vi "DAQ_Power_postwrite.vi"(9 "stop":bool) -> ()   [LabVIEW 2020]
uses:
  <vilib>/Utility/error.llb/DialogType.ctl
  <vilib>/ULx/Create Channel.llb/ULx Create Channel (AI-Voltage-Basic).vi
  <vilib>/ULx/Timing.llb/ULx Timing (Sample Clock).vi
  <vilib>/ULx/Read.llb/ULx Read (Analog 1D Wfm NChan NSamp).vi
panel:
  out "Power Graph":waveform(dbl)[](graph)
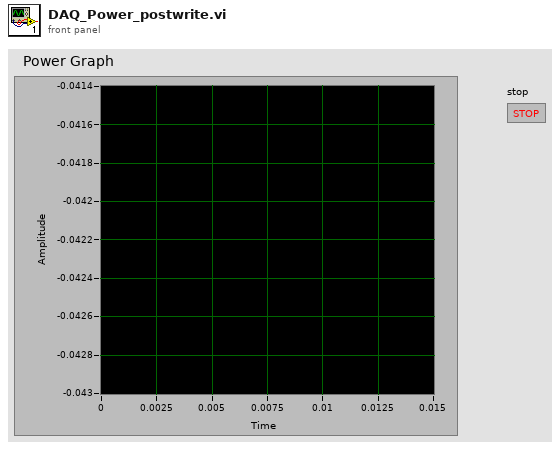
[diagram p1: front panel]
types:
  T1 = typedef "DialogType.ctl" = u16
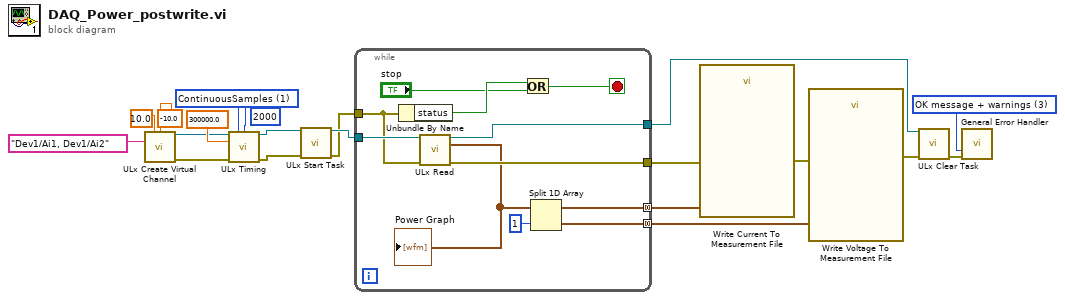
[diagram p0: block diagram]
diagram:
  w16 = 1 items=["FiniteSamples", "ContinuousSamples"] ("sample mode")
  w13 = T1 3 items=["no dialog", "OK message", "continue or stop message", "OK message + warnings", "continue/stop + warnings"] ("type of dialog (OK msg:1)")
  n1 = call-poly <vilib>:"ULx Create Virtual Channel.vi"("maximum value"=10.0, "minimum value"=-10.0, "physical channels"="Dev1/Ai1, Dev1/Ai2") -> ("task out"=w11:refnum<k24>, "error out"=w8:errorcluster)  [unwired: 11 in]
  n2 = call-poly <vilib>:"ULx Timing.vi"("task in"=w11, "sample mode"=w16, "samples per channel"=2000, "rate"=300000.0, "error in"=w8) -> ("task out"=w14:refnum<k24>, "error out"=w15:errorcluster)  [unwired: 9 in]
  n3 = call <vilib>:"ULx Start Task.vi"("task in"=w14, "error in"=w15) -> ("task out"=w12:refnum<k24>, "error out"=w9:errorcluster)  [unwired: 12 in]
  n4 = while {
    tunnel: w9 -> [w27]
    tunnel: w12 -> [w31]
    tunnel: [w30] -> w1
    tunnel: [w25] -> w6
    tunnel: [w22] -> w4 mode=concatenating
    tunnel: [w21] -> w3 mode=concatenating
    stop <- w28 stop-if-true
    n5 = Unbundle By Name(w27) -> ("status"=w29:bool)
    n6 = call-poly <vilib>:"ULx Read.vi"("task in"=w31, "error in"=w27) -> ("task out"=w30:refnum<k24>, "data"=w24:waveform(dbl)[], "error out"=w25:errorcluster)  [unwired: 11 in]
    "Power Graph" <- w24
    n7 = Or(x=w29, y="stop") -> (x .or. y?=w28:bool)
    n8 = Split 1D Array(array=w24, index=1) -> (first subarray=w22:waveform(dbl)[], second subarray=w21:waveform(dbl)[])
  }
  n9 = call "Write Current To Measurement File"("Signals"=w4, "error in (no error)"=w6) -> ("error out"=w2:errorcluster)  [unwired: 15 in, 2 out]
  n10 = call "Write Voltage To Measurement File"("Signals"=w3, "error in (no error)"=w2) -> ("error out"=w5:errorcluster)  [unwired: 15 in, 2 out]
  n11 = call <vilib>:"ULx Clear Task.vi"("task in"=w1, "error in"=w5) -> ("error out"=w10:errorcluster)  [unwired: 13 in]
  n12 = call <vilib>:"General Error Handler.vi"("type of dialog (OK msg:1)"=w13, "error in (no error)"=w10) -> ()  [unwired: 9 in, 5 out]
